vi "AODO-Start Tasks.vi"(0 "AO Tasks":T1[](array[typedef]), 7 "DO Tasks":T2, 11 "error in (no error)":errorcluster) -> (15 "error out":errorcluster)   [LabVIEW 2020]
uses:
  Typedefs/AODO-DO Tasks.ctl
  Typedefs/AODO-Task Specification.ctl
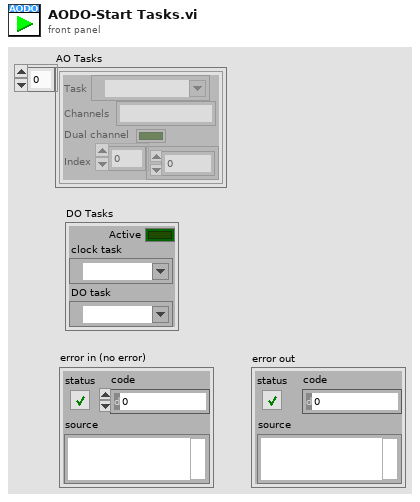
[diagram p1: front panel]
types:
  T1 = typedef "AODO-Task Specification.ctl" = cluster{"Task":refnum<k21>, "Channels":string, "Dual channel":bool, "Index":i32[]}
  T2 = typedef "AODO-DO Tasks.ctl" = cluster{"Active":bool, "clock task":refnum<k21>, "DO task":refnum<k21>}
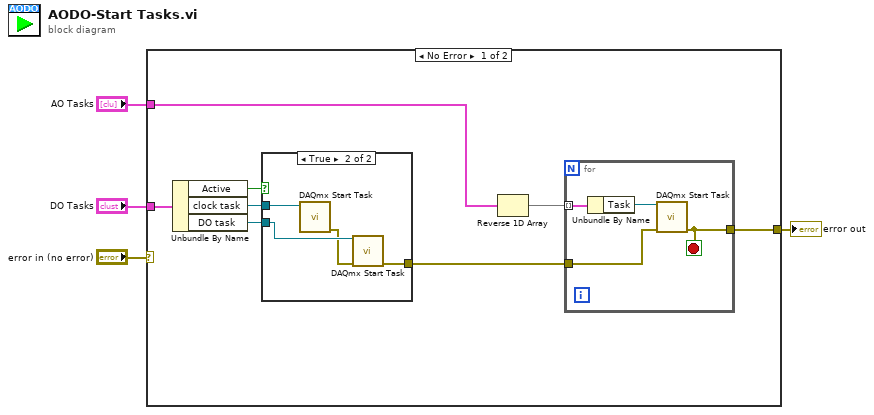
[diagram p0: block diagram]
diagram:
  n1 = case shown="No Error" "error in (no error)" {
    selector: "error in (no error)" -> [_ w21]
    tunnel: "DO Tasks" -> [w11 _]
    tunnel: [w5 w21] -> w3
    tunnel: "AO Tasks" -> [w9 _]
    frame No Error {
      n2 = Unbundle By Name(w11) -> ("Active"=w6:bool, "clock task"=w7:refnum<k21>, "DO task"=w8:refnum<k21>)
      n3 = case shown="True" w6 {
        tunnel: w7 -> [_ w16]
        tunnel: w8 -> [_ w15]
        tunnel: [_ w13] -> w12
        frame False {
        }
        frame True {
          n4 = call <vilib>:"DAQmx Start Task.vi"("task/channels in"=w16) -> ("error out"=w14:errorcluster)  [unwired: 13 in, 1 out]
          n5 = call <vilib>:"DAQmx Start Task.vi"("task/channels in"=w15, "error in"=w14) -> ("error out"=w13:errorcluster)  [unwired: 12 in, 1 out]
        }
      }
      n6 = Reverse 1D Array(array=w9) -> (reversed array=w10:T1[])
      n7 = for {
        tunnel: w10 -> [w20] mode=indexing
        tunnel: [w18] -> w5
        tunnel: w12 -> [w17]
        stop <- w18 stop-if-true
        n8 = Unbundle By Name(w20) -> ("Task"=w19:refnum<k21>)
        n9 = call <vilib>:"DAQmx Start Task.vi"("task/channels in"=w19, "error in"=w17) -> ("error out"=w18:errorcluster)  [unwired: 12 in, 1 out]
      }
    }
    frame Error {
    }
  }
  "error out" <- w3
